vi "Data Generator.vi"(8 "error in (no error)":errorcluster, 11 "Variable Data Type":T1) -> (0 "error out":errorcluster, 3 "Variant":variant)   [LabVIEW 2015]
uses:
  Type Defs/Variable Data Type.ctl
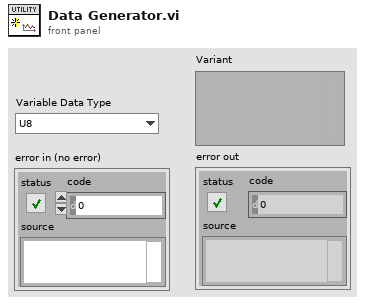
[diagram p1: front panel]
types:
  T1 = typedef "Variable Data Type.ctl" = enum16{"U8", "U16", "U32", "U64", "I8", "I16", "I32", "I64", "Single", "Double", "Boolean", "String"}
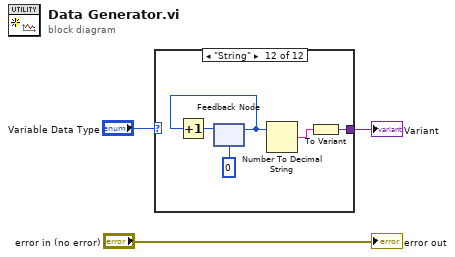
[diagram p0: block diagram]
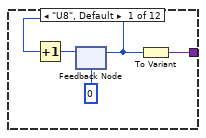
[diagram p2: hidden frame]
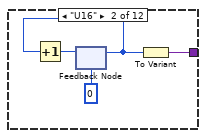
[diagram p3: hidden frame]
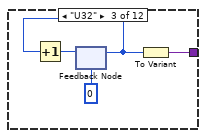
[diagram p4: hidden frame]
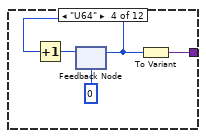
[diagram p5: hidden frame]
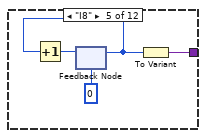
[diagram p6: hidden frame]
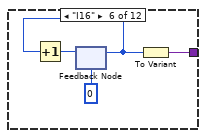
[diagram p7: hidden frame]
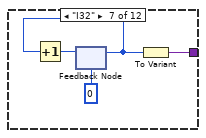
[diagram p8: hidden frame]
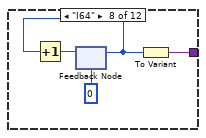
[diagram p9: hidden frame]
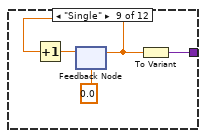
[diagram p10: hidden frame]
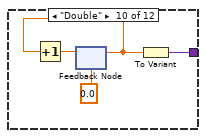
[diagram p11: hidden frame]
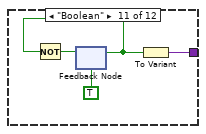
[diagram p12: hidden frame]
diagram:
  n1 = case shown="\"String\"" "Variable Data Type" {
    tunnel: [w4 w8 w12 w16 w20 w24 w28 w32 w36 w40 w44 w51] -> w2
    frame "U8", Default {
      n2 = feedback #1(u8 0) -> (w5:u8)
      n3 = Increment(x=w5) -> (x+1=w6:u8)
      n4 = feedback-in #1(w6) -> ()
      n5 = To Variant(anything=w5) -> (Variant=w4:variant)
    }
    frame "U16" {
      n6 = feedback #2(u16 0) -> (w9:u16)
      n7 = Increment(x=w9) -> (x+1=w10:u16)
      n8 = feedback-in #2(w10) -> ()
      n9 = To Variant(anything=w9) -> (Variant=w8:variant)
    }
    frame "U32" {
      n10 = feedback #3(u32 0) -> (w13:u32)
      n11 = Increment(x=w13) -> (x+1=w14:u32)
      n12 = feedback-in #3(w14) -> ()
      n13 = To Variant(anything=w13) -> (Variant=w12:variant)
    }
    frame "U64" {
      n14 = feedback #4(u64 0) -> (w17:u64)
      n15 = Increment(x=w17) -> (x+1=w18:u64)
      n16 = feedback-in #4(w18) -> ()
      n17 = To Variant(anything=w17) -> (Variant=w16:variant)
    }
    frame "I8" {
      n18 = feedback #5(i8 0) -> (w21:i8)
      n19 = Increment(x=w21) -> (x+1=w22:i8)
      n20 = feedback-in #5(w22) -> ()
      n21 = To Variant(anything=w21) -> (Variant=w20:variant)
    }
    frame "I16" {
      n22 = feedback #6(i16 0) -> (w25:i16)
      n23 = Increment(x=w25) -> (x+1=w26:i16)
      n24 = feedback-in #6(w26) -> ()
      n25 = To Variant(anything=w25) -> (Variant=w24:variant)
    }
    frame "I32" {
      n26 = feedback #7(0) -> (w29:i32)
      n27 = Increment(x=w29) -> (x+1=w30:i32)
      n28 = feedback-in #7(w30) -> ()
      n29 = To Variant(anything=w29) -> (Variant=w28:variant)
    }
    frame "I64" {
      n30 = feedback #8(i64 0) -> (w33:i64)
      n31 = Increment(x=w33) -> (x+1=w34:i64)
      n32 = feedback-in #8(w34) -> ()
      n33 = To Variant(anything=w33) -> (Variant=w32:variant)
    }
    frame "Single" {
      n34 = feedback #9(sgl 0.0) -> (w37:sgl)
      n35 = Increment(x=w37) -> (x+1=w38:sgl)
      n36 = feedback-in #9(w38) -> ()
      n37 = To Variant(anything=w37) -> (Variant=w36:variant)
    }
    frame "Double" {
      n38 = feedback #10(0.0) -> (w41:dbl)
      n39 = Increment(x=w41) -> (x+1=w42:dbl)
      n40 = feedback-in #10(w42) -> ()
      n41 = To Variant(anything=w41) -> (Variant=w40:variant)
    }
    frame "Boolean" {
      n42 = feedback #11(TRUE) -> (w45:bool)
      n43 = Not(x=w45) -> (.not. x?=w46:bool)
      n44 = feedback-in #11(w46) -> ()
      n45 = To Variant(anything=w45) -> (Variant=w44:variant)
    }
    frame "String" {
      n46 = feedback #12(0) -> (w49:i32)
      n47 = Increment(x=w49) -> (x+1=w52:i32)
      n48 = feedback-in #12(w52) -> ()
      n49 = Number To Decimal String(number=w49) -> (decimal integer string=w48:string)  [unwired: 1 in]
      n50 = To Variant(anything=w48) -> (Variant=w51:variant)
    }
  }
  "Variant" <- w2
  "error out" <- "error in (no error)"
